vi "picoReady.vi"(8 "error in (no error)":errorcluster, 11 "handle in":i16) -> (0 "error out":errorcluster, 3 "handle out":i16)   [LabVIEW 2011]
uses:
  PS2000a.dll
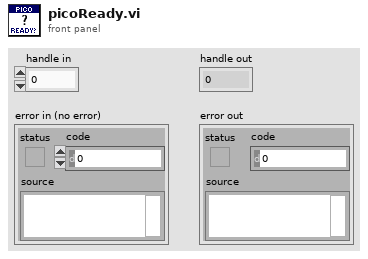
[diagram p1: front panel]
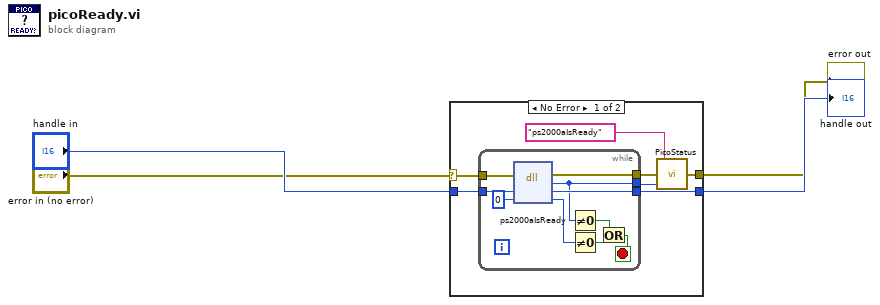
[diagram p0: block diagram]
diagram:
  n1 = case shown="No Error" "error in (no error)" {
    selector: "error in (no error)" -> [w9 w22]
    tunnel: "handle in" -> [w11 w23]
    tunnel: [w10 w23] -> w4
    tunnel: [w8 w22] -> w3
    frame No Error {
      n2 = while {
        tunnel: [w21] -> w10
        tunnel: w11 -> [w20]
        tunnel: [w15] -> w6
        tunnel: w9 -> [w14]
        tunnel: [w13] -> w7
        stop <- w19 stop-if-true
        n3 = dll-call lib="ps2000a.dll" fn="ps2000aIsReady" ("ps3000.dll:_ps3000_open_unit@0")(error in=w14, "handle"=w20, "ready"=i16 0) -> (error out=w13:errorcluster, "status"=w15:i32, "handle"=w21:i16, "ready"=w16:i16)  [unwired: 2 in, 1 out]
        n4 = Not Equal To 0?(x=w15) -> (x != 0?=w17:bool)
        n5 = Not Equal To 0?(x=w16) -> (x != 0?=w18:bool)
        n6 = Or(x=w17, y=w18) -> (x .or. y?=w19:bool)
      }
      n7 = call "PicoStatus.vi"("PICO STATUS"=w6, "error in"=w7, "source"="ps2000aIsReady") -> ("error out"=w8:errorcluster)
    }
    frame Error {
    }
  }
  "handle out" <- w4
  "error out" <- w3
